vi "rethinkdb_tcp_pop_message.vi"(8 "error in (no error)":errorcluster, 9 "offset (0)":i32, 10 "data in":string) -> (0 "error out":errorcluster, 1 "offset past match":i32, 2 "unterminated?":bool, 3 "next message":string)   [LabVIEW 2017]
uses:
  <vilib>/Utility/error.llb/Error Cluster From Error Code.vi
  <vilib>/ErrorRing/Error Ring.xnode
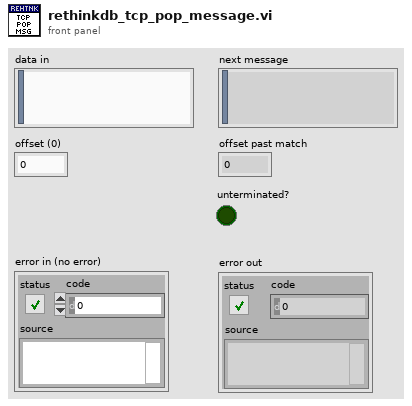
[diagram p1: front panel]
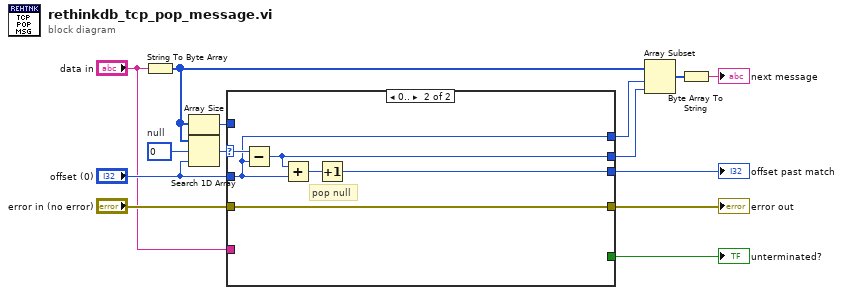
[diagram p0: block diagram]
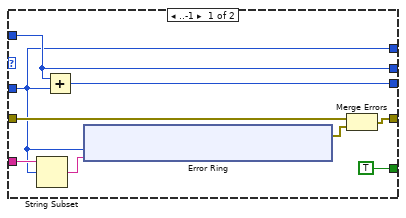
[diagram p2: hidden frame]
diagram:
  w14 = u8 0  # null
  n1 = String To Byte Array(string="data in") -> (unsigned byte array=w9:u8[])
  n2 = Array Size(array=w9) -> (size(s)=w8:i32)
  n3 = Search 1D Array(1D array=w9, element=w14, start index (0)="offset (0)") -> (index of element=w11:i32)
  n4 = case shown="0.." w11 {
    selector: w11 -> [_ w37]
    tunnel: "offset (0)" -> [w16 w34]
    tunnel: [w17 w35] -> w6
    tunnel: [w16 w34] -> w7
    tunnel: w8 -> [w17 _]
    tunnel: [w20 w36] -> w5
    tunnel: "error in (no error)" -> [w23 w36]
    tunnel: "data in" -> [w22 _]
    tunnel: [TRUE _] -> w2
    tunnel: [w15 w32] -> w1
    frame ..-1 {
      n5 = String Subset(string=w22, offset (0)=w16) -> (substring=w21:string)  [unwired: 1 in]
      n6 = Add(x=w17, y=w16) -> (x+y=w15:i32)
      n7 = xnode "Error Ring"("parameter 0"=w16, "parameter 1"=w21) -> ("error out"=w19:errorcluster)
      n8 = Merge Errors(w23, w19) -> (w20:errorcluster)
    }
    frame 0.. {
      # "pop null"
      n9 = Subtract(x=w37, y=w34) -> (x-y=w35:i32)
      n10 = Add(x=w35, y=w34) -> (x+y=w33:i32)
      n11 = Increment(x=w33) -> (x+1=w32:i32)
    }
  }
  "unterminated?" <- w2
  "offset past match" <- w1
  "error out" <- w5
  n12 = Array Subset(array=w9, index=w7, length=w6) -> (w13:u8[])
  n13 = Byte Array To String(unsigned byte array=w13) -> (string=→"next message":string)
